vi "loadingCircle.vi"() -> ()   [LabVIEW 2015]
uses:
  <vilib>/Utility/miscctls.llb/LVBoundsTypeDef.ctl
panel:
  in  "Round Color Box 12":u32(colorbox)
  in  "Round Color Box 11":u32(colorbox)
  in  "Round Color Box 10":u32(colorbox)
  in  "Round Color Box 9":u32(colorbox)
  in  "Round Color Box 8":u32(colorbox)
  in  "Round Color Box 7":u32(colorbox)
  in  "Round Color Box 6":u32(colorbox)
  in  "Round Color Box 5":u32(colorbox)
  in  "Round Color Box 4":u32(colorbox)
  in  "Round Color Box 3":u32(colorbox)
  in  "Round Color Box 2":u32(colorbox)
  in  "Round Color Box":u32(colorbox)
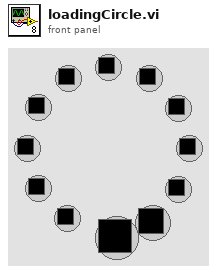
[diagram p1: front panel]
types:
  T1 = typedef "LVBoundsTypeDef.ctl" = cluster{"Width":u32, "Height":u32}
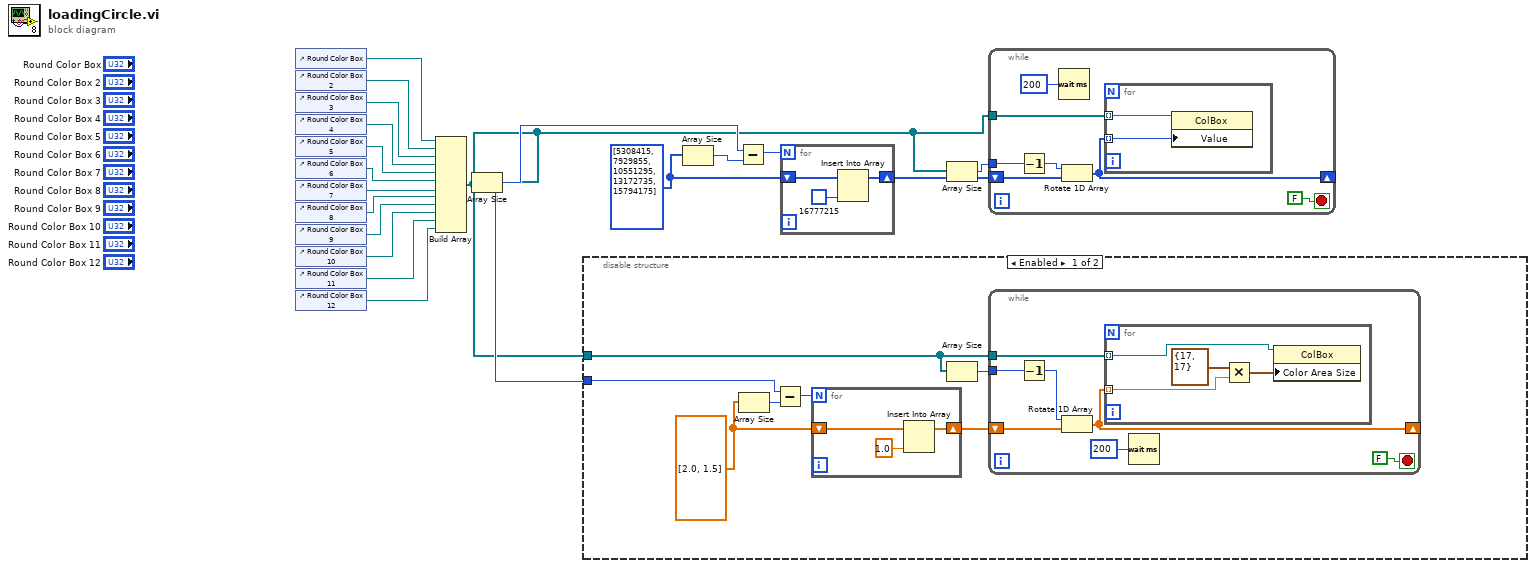
[diagram p0: block diagram]
diagram:
  w8 = u32[] [5308415, 7929855, 10551295, 13172735, 15794175]
  n1 = control-ref of="Round Color Box"() -> (w19:refnum<vi>)
  n2 = control-ref of="Round Color Box 2"() -> (w18:refnum<vi>)
  n3 = control-ref of="Round Color Box 3"() -> (w17:refnum<vi>)
  n4 = control-ref of="Round Color Box 4"() -> (w1:refnum<vi>)
  n5 = control-ref of="Round Color Box 5"() -> (w16:refnum<vi>)
  n6 = control-ref of="Round Color Box 6"() -> (w15:refnum<vi>)
  n7 = control-ref of="Round Color Box 7"() -> (w14:refnum<vi>)
  n8 = control-ref of="Round Color Box 8"() -> (w13:refnum<vi>)
  n9 = control-ref of="Round Color Box 9"() -> (w12:refnum<vi>)
  n10 = control-ref of="Round Color Box 10"() -> (w11:refnum<vi>)
  n11 = control-ref of="Round Color Box 11"() -> (w10:refnum<vi>)
  n12 = control-ref of="Round Color Box 12"() -> (w9:refnum<vi>)
  n13 = Build Array(w19, w18, w17, w1, w16, w15, w14, w13, w12, w11, w10, w9) -> (w2:refnum<vi>[])
  n14 = Array Size(array=w2) -> (size(s)=w5:i32)
  n15 = disable-structure shown="Enabled" {
    disable-tunnel: w5 -> [w24 _]
    disable-tunnel: w2 -> [w20 _]
    frame Enabled {
      w22 = dbl[] [2.0, 1.5]
      n16 = Array Size(array=w22) -> (size(s)=w23:i32)
      n17 = Subtract(x=w24, y=w23) -> (x-y=w25:i32)
      n18 = for {
        N: w25 -> [_]
        shift-right: [w27] -> w26
        shift-left: w22 -> [w28]
        n19 = Insert Into Array(array=w28, new element=1.0) -> (w27:dbl[])  [unwired: 1 in]
      }
      n20 = Array Size(array=w20) -> (size(s)=w21:i32)
      n21 = while {
        tunnel: w20 -> [w34]
        shift-right: [w32] -> _
        shift-left: w26 -> [w33]
        tunnel: w21 -> [w30]
        stop <- FALSE stop-if-true
        n22 = Decrement(x=w30) -> (x-1=w31:i32)
        n23 = Rotate 1D Array(1:w33, 2:w31) -> (0:w32:dbl[])
        n24 = for {
          tunnel: w34 -> [w40] mode=indexing
          tunnel: w32 -> [w39] mode=indexing
          n25 = Multiply(x=T1 {"Width"=17, "Height"=17} ("Color Area Size"), y=w39) -> (x*y=w37:cluster{"Width":dbl, "Height":dbl})
          n26 = property class="ColBox"(reference=w40, "Color Area Size"=w37) -> ()  [unwired: 1 in, 2 out]
        }
        n27 = Wait (ms)(milliseconds to wait=u32 200) -> ()  [unwired: 1 out]
      }
    }
    frame Disabled {
    }
  }
  n28 = Array Size(array=w8) -> (size(s)=w7:i32)
  n29 = Subtract(x=w5, y=w7) -> (x-y=w6:i32)
  n30 = for {
    N: w6 -> [_]
    shift-right: [w42] -> w4
    shift-left: w8 -> [w43]
    n31 = Insert Into Array(array=w43, new element=u32 16777215 ("Round Color Box")) -> (w42:u32[])  [unwired: 1 in]
  }
  n32 = Array Size(array=w2) -> (size(s)=w3:i32)
  n33 = while {
    shift-right: [w47] -> _
    shift-left: w4 -> [w50]
    tunnel: w3 -> [w46]
    tunnel: w2 -> [w44]
    stop <- FALSE stop-if-true
    n34 = Decrement(x=w46) -> (x-1=w45:i32)
    n35 = Wait (ms)(milliseconds to wait=u32 200) -> ()  [unwired: 1 out]
    n36 = Rotate 1D Array(1:w50, 2:w45) -> (0:w47:u32[])
    n37 = for {
      tunnel: w47 -> [w52] mode=indexing
      tunnel: w44 -> [w51] mode=indexing
      n38 = property class="ColBox"(reference=w51, "Value"=w52) -> ()  [unwired: 1 in, 2 out]
    }
  }
